vi "SN Sort Data.vi"(7 "Array In":string[][](array[string])) -> (8 "Array Out":string[][](array[string]), 15 "EarliestDate":string)   [LabVIEW 2013]
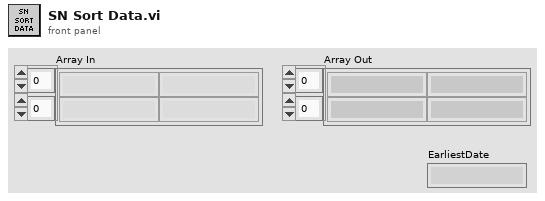
[diagram p1: front panel]
types:
  T1 = cluster{"Sortable Date":string, string, string, string, string, "Array In":string[]}
  T2 = cluster{"Sortable Date":string, string, string, string, string, "Array In":string[]}[]
  T3 = cluster{string, string, string, string, "Sortable Date":string, "Array In":string[]}
  T4 = cluster{string, string, string, string, "Sortable Date":string, "Array In":string[]}[]
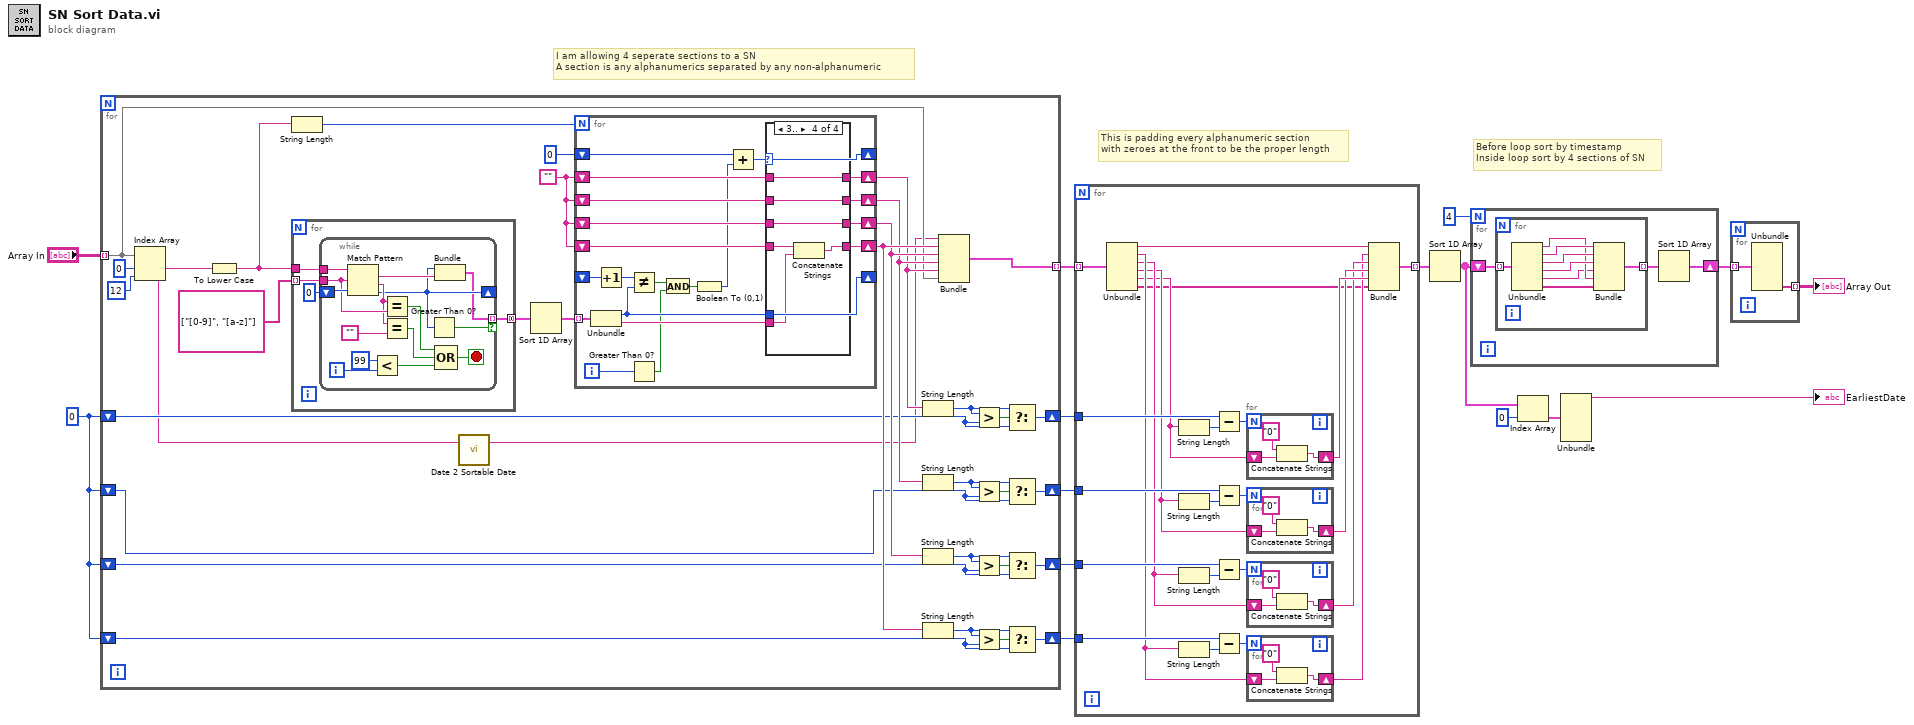
[diagram p0: block diagram]
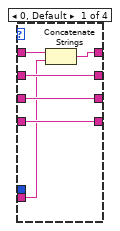
[diagram p2: hidden frame]
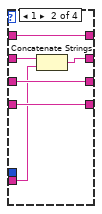
[diagram p3: hidden frame]
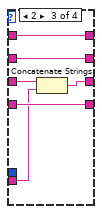
[diagram p4: hidden frame]
diagram:
  w14 = 0
  # "Before loop sort by timestamp\nInside loop sort by 4 sections of SN"
  # "This is padding every alphanumeric section\nwith zeroes at the front to be the proper length"
  # "I am allowing 4 seperate sections to a SN\nA section is any alphanumerics separated by any non-alphanumeric"
  n1 = for {
    tunnel: [w42] -> w15 mode=indexing
    tunnel: "Array In" -> [w17] mode=indexing
    shift-right: [w28] -> w12
    shift-left: w14 -> [w19]
    shift-right: [w26] -> w11
    shift-left: w14 -> [w30]
    shift-right: [w27] -> w10
    shift-left: w14 -> [w29]
    shift-right: [w34] -> w13
    shift-left: w14 -> [w35]
    w43 = ""
    n2 = Index Array(array=w17, index #1=0 ("index"), index #2=12 ("index")) -> (element #1=w22:string, element #2=w18:string)
    n3 = To Lower Case(string=w22) -> (all lower case string=w48:string)
    n4 = String Length(string=w48) -> (length=w45:i32)
    n5 = for {
      tunnel: string[] ["[0-9]", "[a-z]"] -> [w96] mode=indexing
      tunnel: w48 -> [w97]
      tunnel: [w94] -> w47 mode=concatenating
      n6 = while {
        tunnel: w97 -> [w112]
        tunnel: w96 -> [w107]
        shift-right: [w99] -> _
        shift-left: 0 ("offset past match") -> [w111]
        tunnel: [w98] -> w94 mode=indexing if=w101
        i -> [w109]
        stop <- w102 stop-if-true
        n7 = Match Pattern(string=w112, regular expression=w107, offset (0)=w111) -> (match substring=w100:string, after substring=w106:string, offset past match=w99:i32)  [unwired: 1 out]
        n8 = Less?(x=99, y=w109) -> (x < y?=w108:bool)
        n9 = Equal?(x=w106, y=w107) -> (x = y?=w103:bool)
        n10 = Equal?(x=w106, y="") -> (x = y?=w104:bool)
        n11 = Greater Than 0?(x=w99) -> (x > 0?=w101:bool)
        n12 = Bundle("offset past match"=w99, w100) -> (w98:cluster{"offset past match":i32, string})  [unwired: 1 in]
        n13 = Compound Arithmetic op=OR(w103, w104, w108) -> (w102:bool)
      }
    }
    n14 = call "Date 2 Sortable Date.vi"("Date String"=w18) -> ("Sortable Date"=w16:string)  [unwired: 2 in]
    n15 = Sort 1D Array(array=w47) -> (sorted array=w46:cluster{"offset past match":i32, string}[])
    n16 = for {
      N: w45 -> [_]
      tunnel: w46 -> [w69] mode=indexing
      shift-right: [w55] -> _
      shift-left: 0 -> [w56]
      shift-right: [w61] -> w38
      shift-left: w43 -> [w68]
      shift-right: [w64] -> w39
      shift-left: w43 -> [w67]
      shift-right: [w63] -> w40
      shift-left: w43 -> [w66]
      shift-right: [w62] -> w41
      shift-left: w43 -> [w65]
      shift-right: [w58] -> _
      shift-left: _ -> [w60]
      i -> [w51]
      n17 = Unbundle(w69) -> ("offset past match"=w58:i32, w54:string)
      n18 = Increment(x=w60) -> (x+1=w59:i32)
      n19 = Not Equal?(x=w59, y=w58) -> (x != y?=w53:bool)
      n20 = Greater Than 0?(x=w51) -> (x > 0?=w52:bool)
      n21 = And(x=w53, y=w52) -> (x .and. y?=w50:bool)
      n22 = Boolean To (0,1)(Boolean=w50) -> (0, 1=w57:i16)
      n23 = Add(x=w56, y=w57) -> (x+y=w55:i32)
      n24 = case shown="3.." w55 {
        tunnel: w58 -> [_ _ _ _]
        tunnel: w68 -> [w72 w77 w86 w93]
        tunnel: w67 -> [w75 w79 w83 w92]
        tunnel: w66 -> [w74 w81 w85 w90]
        tunnel: w65 -> [w73 w80 w87 w91]
        tunnel: [w75 w78 w83 w92] -> w64
        tunnel: [w74 w81 w84 w90] -> w63
        tunnel: [w73 w80 w87 w89] -> w62
        tunnel: [w71 w77 w86 w93] -> w61
        tunnel: w54 -> [w70 w76 w82 w88]
        frame 0, Default {
          n25 = Concatenate Strings(w72, w70) -> (w71:string)
        }
        frame 1 {
          n26 = Concatenate Strings(w79, w76) -> (w78:string)
        }
        frame 2 {
          n27 = Concatenate Strings(w85, w82) -> (w84:string)
        }
        frame 3.. {
          n28 = Concatenate Strings(w91, w88) -> (w89:string)
        }
      }
    }
    n29 = String Length(string=w38) -> (length=w37:i32)
    n30 = String Length(string=w39) -> (length=w25:i32)
    n31 = String Length(string=w40) -> (length=w24:i32)
    n32 = String Length(string=w41) -> (length=w23:i32)
    n33 = Bundle("Sortable Date"=w16, w41, w40, w39, w38, "Array In"=w17) -> (w42:T1)  [unwired: 1 in]
    n34 = Greater?(x=w37, y=w35) -> (0:w36:bool)
    n35 = Greater?(x=w25, y=w19) -> (0:w31:bool)
    n36 = Greater?(x=w24, y=w30) -> (0:w33:bool)
    n37 = Greater?(x=w23, y=w29) -> (0:w32:bool)
    n38 = Select(t=w37, s=w36, f=w35) -> (s? t:f=w34:i32)
    n39 = Select(t=w25, s=w31, f=w19) -> (s? t:f=w28:i32)
    n40 = Select(t=w24, s=w33, f=w30) -> (s? t:f=w26:i32)
    n41 = Select(t=w23, s=w32, f=w29) -> (s? t:f=w27:i32)
  }
  n42 = for {
    tunnel: w15 -> [w116] mode=indexing
    tunnel: w12 -> [w131]
    tunnel: w13 -> [w136]
    tunnel: w11 -> [w126]
    tunnel: w10 -> [w125]
    tunnel: [w120] -> w7 mode=indexing
    n43 = Unbundle(w116) -> ("Sortable Date"=w113:string, w119:string, w118:string, w117:string, w115:string, "Array In"=w114:string[])
    n44 = String Length(string=w115) -> (length=w135:i32)
    n45 = String Length(string=w117) -> (length=w132:i32)
    n46 = String Length(string=w118) -> (length=w127:i32)
    n47 = String Length(string=w119) -> (length=w130:i32)
    n48 = Subtract(x=w136, y=w135) -> (x-y=w134:i32)
    n49 = Subtract(x=w131, y=w132) -> (x-y=w133:i32)
    n50 = Subtract(x=w126, y=w127) -> (x-y=w128:i32)
    n51 = Subtract(x=w125, y=w130) -> (x-y=w129:i32)
    n52 = for {
      N: w134 -> [_]
      shift-right: [w147] -> w124
      shift-left: w115 -> [w148]
      n53 = Concatenate Strings("0", w148) -> (w147:string)
    }
    n54 = for {
      N: w133 -> [_]
      shift-right: [w144] -> w123
      shift-left: w117 -> [w145]
      n55 = Concatenate Strings("0", w145) -> (w144:string)
    }
    n56 = for {
      N: w128 -> [_]
      shift-right: [w141] -> w122
      shift-left: w118 -> [w142]
      n57 = Concatenate Strings("0", w142) -> (w141:string)
    }
    n58 = for {
      N: w129 -> [_]
      shift-right: [w138] -> w121
      shift-left: w119 -> [w139]
      n59 = Concatenate Strings("0", w139) -> (w138:string)
    }
    n60 = Bundle("Sortable Date"=w113, w121, w122, w123, w124, "Array In"=w114) -> (w120:T1)  [unwired: 1 in]
  }
  n61 = Sort 1D Array(array=w7) -> (sorted array=w2:T2)
  n62 = for {
    N: 4 -> [_]
    shift-right: [w149] -> w8
    shift-left: w2 -> [w151]
    n63 = for {
      tunnel: w151 -> [w159] mode=indexing
      tunnel: [w158] -> w150 mode=indexing
      n64 = Unbundle(w159) -> ("Sortable Date"=w153:string, w155:string, w156:string, w157:string, w152:string, "Array In"=w154:string[])
      n65 = Bundle(w155, w156, w157, w152, "Sortable Date"=w153, "Array In"=w154) -> (w158:T3)  [unwired: 1 in]
    }
    n66 = Sort 1D Array(array=w150) -> (sorted array=w149:T4)
  }
  n67 = Index Array(array=w2, index=0) -> (element=w3:T1)
  n68 = Unbundle(w3) -> ("Sortable Date"=→"EarliestDate":string)  [unwired: 5 out]
  n69 = for {
    tunnel: w8 -> [w161] mode=indexing
    tunnel: [w160] -> w5 mode=indexing
    n70 = Unbundle(w161) -> ("Array In"=w160:string[])  [unwired: 5 out]
  }
  "Array Out" <- w5
